vi "Get Audio File Info.vi"   [LabVIEW 2020, in "G-Audio.lvlib"]
doc: "Retrieve audio file information. Some codecs (mp3) require the entire file be parsed to accurately determine the length, which can take time for very large files.\n\nSupported codecs: flac, mp3, ogg (vorbis), and wav."
uses:
  G-Audio.lvlib
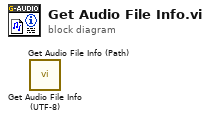
[diagram p0: block diagram]
diagram:
  n1 = call "Get Audio File Info (UTF-8).vi"() -> ()  [unwired: 7 in, 5 out]
  n2 = call "Get Audio File Info (Path).vi"() -> ()  [unwired: 7 in, 5 out]
